vi "Initialization.vi"(8 "error in":errorcluster, 10 "Acc_delay":u16, 11 "FPGA VI Reference In":T2) -> (0 "error out":errorcluster, 3 "FPGA VI Reference Out":T1)   [LabVIEW 2025]
uses:
  FPGA_ref_in.ctl
  FPGA_ref_out.ctl
  <vilib>/Utility/error.llb/Error Cluster From Error Code.vi
  <vilib>/rvi/errors/niLvFpgaAdjustHostInterfaceError.vi
  <vilib>/rvi/interface/common/niFpgaWaitOnOcc.vi
  <vilib>/FPGAPlugInAG/Dynamic/niLvFpga_Run_Dynamic.vi
  <vilib>/rvi/interface/nirviReadWriteControl/nirviReadWriteControl.xnode
  <vilib>/rvi/interface/nirviMethod/nirviMethod.xnode
  <vilib>/FPGAPlugInAG/Dynamic/niLvFpga_ConfigureFifo_Dynamic.vi
  <vilib>/rvi/errors/niLvFpgaMergeErrorWithErrorCode.vi
  NiFpgaLv.dll
  <vilib>/rvi/interface/Simulation/niFpgaSimulationCallBeginRW.vi
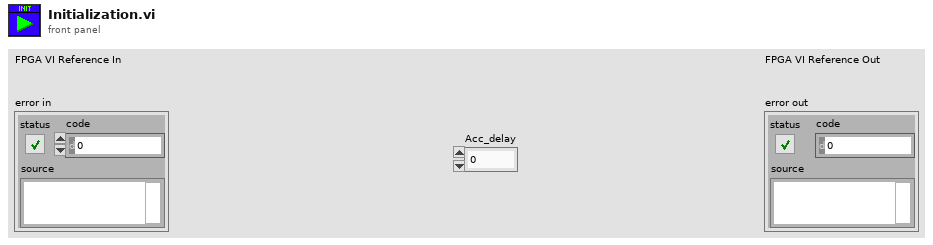
[diagram p1: front panel]
types:
  T1 = typedef "FPGA_ref_out.ctl" = refnum<k20>
  T2 = typedef "FPGA_ref_in.ctl" = refnum<k20>
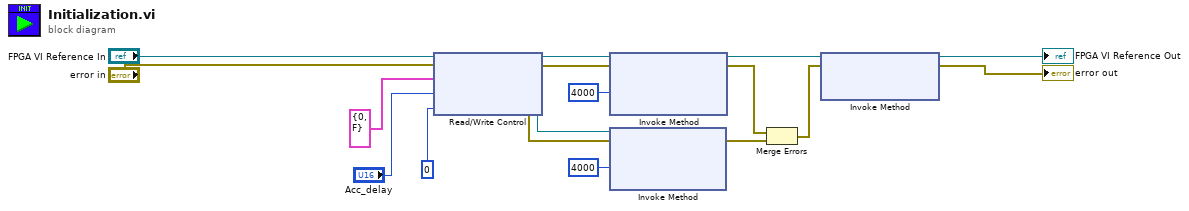
[diagram p0: block diagram]
diagram:
  n1 = xnode "Read/Write Control"("FPGA VI Reference In"="FPGA VI Reference In", "error in"="error in", "Var data"=cluster{"Placeholder":i16, "Trigger":bool} {"Placeholder"=0, "Trigger"=FALSE}, "Time Delay_Read"="Acc_delay", "Time delay_Send"=u16 0 ("SENDCount(uSec) 2")) -> ("FPGA VI Reference Out"=w6:T2, "error out"=w4:errorcluster)
  n2 = xnode "Invoke Method"("FPGA VI Reference In"=w6, "error in"=w4, "Requested Depth"=u32 4000) -> ("FPGA VI Reference Out"=w13:T2, "error out"=w11:errorcluster)  [unwired: 1 out]
  n3 = xnode "Invoke Method"("FPGA VI Reference In"=w6, "error in"=w4, "Requested Depth"=u32 4000) -> ("error out"=w10:errorcluster)  [unwired: 2 out]
  n4 = Merge Errors(w11, w10) -> (w12:errorcluster)
  n5 = xnode "Invoke Method"("FPGA VI Reference In"=w13, "error in"=w12) -> ("FPGA VI Reference Out"=→"FPGA VI Reference Out":T2, "error out"=→"error out":errorcluster)  [unwired: 1 in]
